vi "_PC_Daemon_DisInstrumentParam.vi"(8 "error in":errorcluster, 11 "ExpCondi":T1=[{"Label"="Laser", "Value"=variant}, {"Label"="Pressure", "Value"=variant}, {"Label"="TMP", "Value"=variant}, {"Label"="Script", "Value"=variant}, {"Label"="Signal Remarks", "Value"=variant}, {"Label"="ExtAO", "Value"=variant}, {"Label"="ExtDO", "Value"=variant}, {"Label"="ExtDI", "Value"=variant}, {"Label"="D999", "Value"=variant}]) -> (0 "error out":errorcluster)   [LabVIEW 2018]
uses:
  RT/PublicSubVI/Ctl/_ctl_RT_ExpCondi.ctl
  <vilib>/Utility/miscctls.llb/LVRowAndColumnTypeDef.ctl
  <vilib>/Utility/miscctls.llb/LVRowAndColumnUnsignedTypeDef.ctl
  <vilib>/event_ctls.llb/eventvkey.ctl
  PublicSubVI/Ctl/RegistyFunc.ctl
  <vilib>/Utility/file.llb/Write Delimited Spreadsheet (string).vi
panel:
  in  "Close Button":bool
  in  "Export Button":bool
  out "Table":string[][](table)
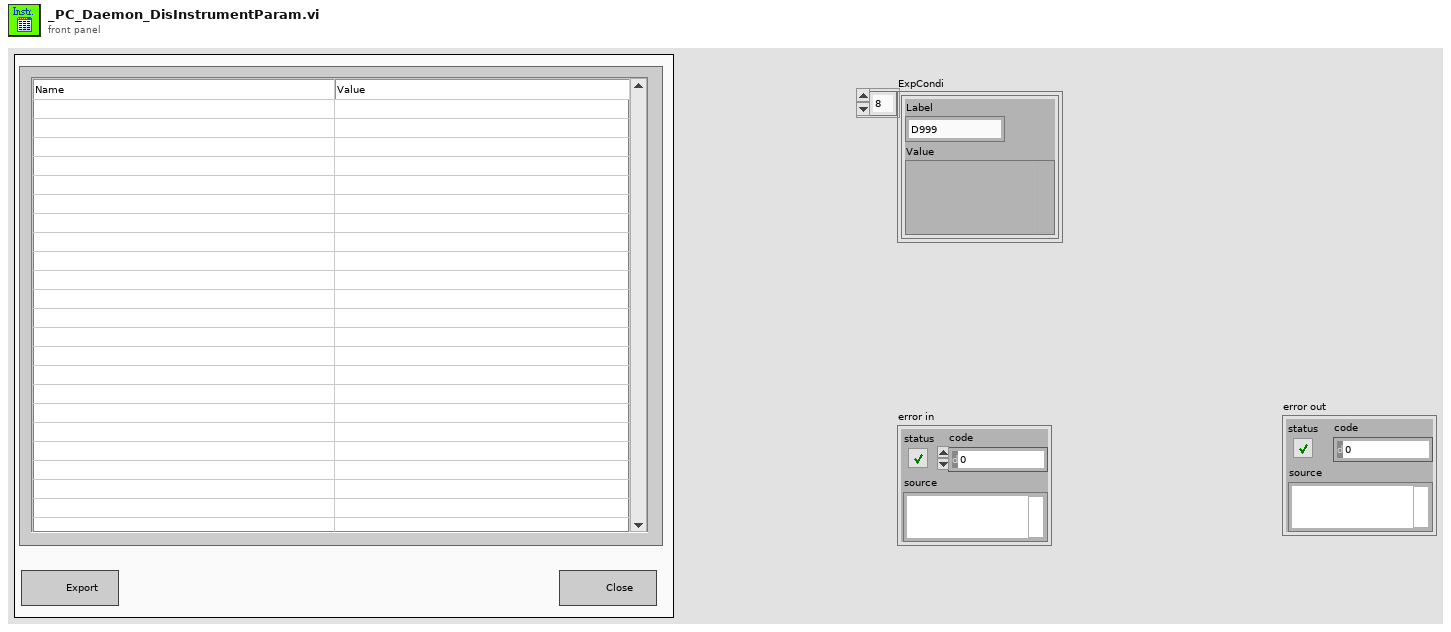
[diagram p1: front panel]
types:
  T1 = typedef "_ctl_RT_ExpCondi.ctl" = cluster{"Label":string, "Value":variant}[]
  T2 = typedef "LVRowAndColumnUnsignedTypeDef.ctl" = cluster{"Row":u32, "Column":u32}
  T3 = typedef "LVRowAndColumnTypeDef.ctl" = cluster{"Row":i32, "Column":i32}
  T4 = typedef "eventvkey.ctl" = enum16{"ASCII", "Enter", "Return", "Shift", "Ctrl", "Alt", "Cmd", "Opt", "Caps", "NumLock", "Clear", "Break", "Up", "Down", "Left", "Right", "Insert", "Delete", "Home", "End", "PageUp", "PageDown", "Escape", "Help", "Pause", "ScrollLock", "F1", "F2", "F3", "F4", "F5", "F6", "F7", "F8", "F9", "F10", "F11", "F12", "F13", "F14", "F15", "F16", "F17", "F18", "F19", "F20", "F21", "F22", "F23", "F24", "Play", "VolumeUp", "VolumeDown", "Mute", "Two Byte Char"}
  T5 = typedef "RegistyFunc.ctl" = enum16{"None", "FileAutoSave", "FileNoise", "FileSN", "ExeStatu", "WorkFolderPath", "MethodPath", "AVGItem", "LoopItem", "AutoRun", "BGColor", "LineColor", "LineWidth", "XGrid", "YGrid", "DeviceRefnum"}
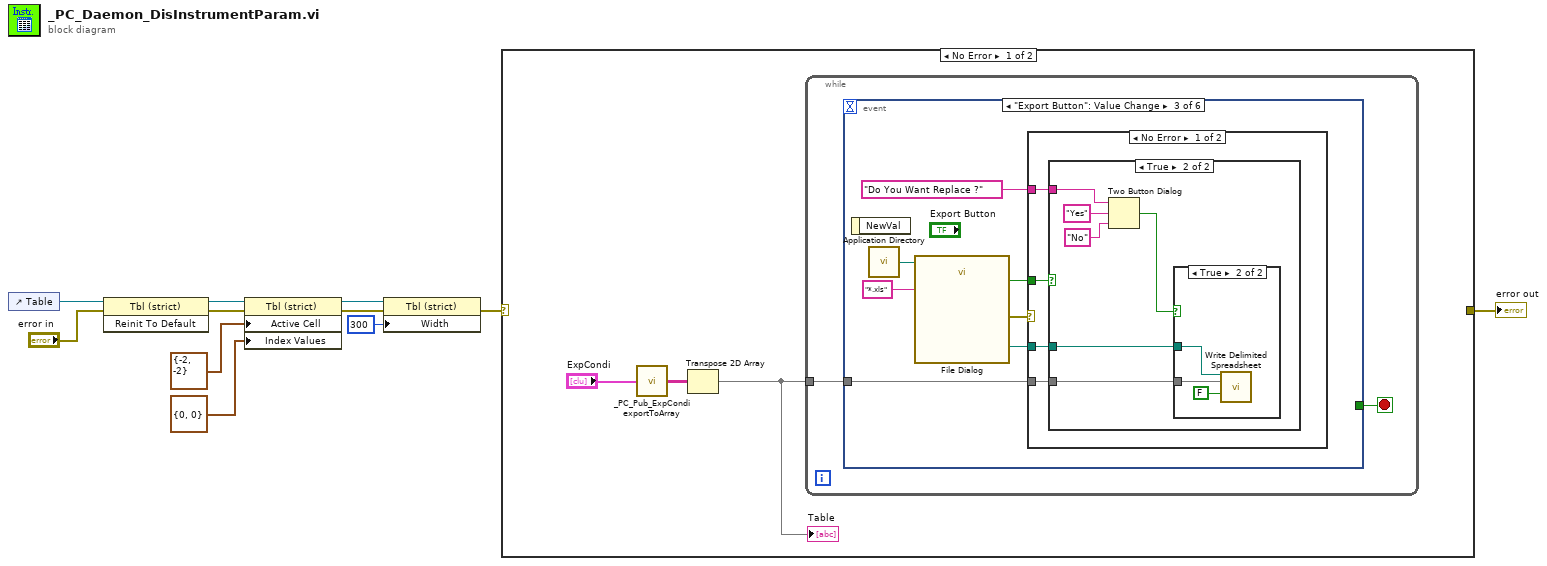
[diagram p0: block diagram]
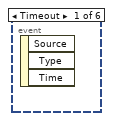
[diagram p2: hidden frame]
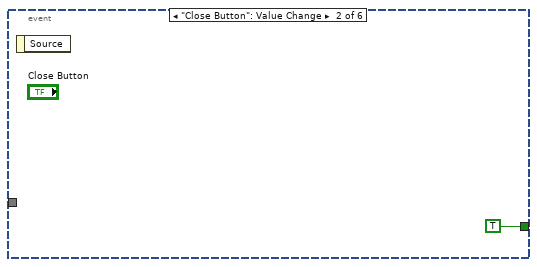
[diagram p3: hidden frame]
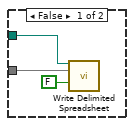
[diagram p4: hidden frame]
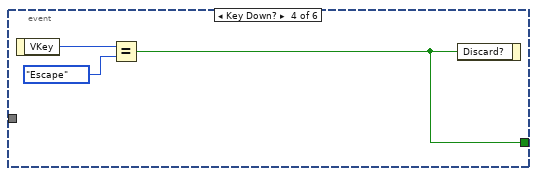
[diagram p7: hidden frame]
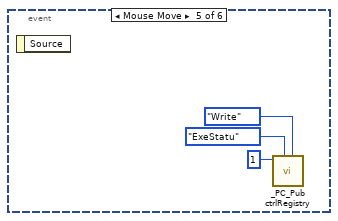
[diagram p8: hidden frame]
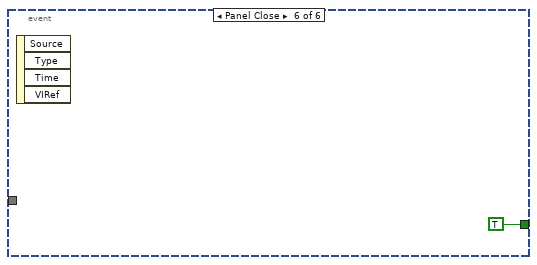
[diagram p9: hidden frame]
diagram:
  n1 = control-ref of="Table"() -> (w6:refnum<vi>)
  n2 = invoke class="Tbl (strict)" method="Reinit To Default"(reference=w6, error in="error in") -> (reference out=w5:refnum<vi>, error out=w4:errorcluster)  [unwired: 1 in, 1 out]
  n3 = property class="Tbl (strict)"(reference=w5, error in=w4, "Active Cell"=T3 {"Row"=-2, "Column"=-2} ("Active Cell:Active Cell"), "Index Values"=T2 {"Row"=0, "Column"=0}) -> (reference out=w9:refnum<vi>, error out=w8:errorcluster)
  n4 = property class="Tbl (strict)"(reference=w9, error in=w8, "Width"=u32 300 ("Active Cell:Cell Size:Width")) -> (error out=w2:errorcluster)  [unwired: 1 out]
  n5 = case shown="No Error" w2 {
    selector: w2 -> [_ w48]
    tunnel: [_ w48] -> w1
    frame No Error {
      n6 = call "_PC_Pub_ExpCondi exportToArray.vi"("ExpCondi"="ExpCondi") -> ("appended array"=w14:string[][])
      n7 = Transpose 2D Array(2D array=w14) -> (transposed array=w13:string[][])
      "Table" <- w13
      n8 = while {
        tunnel: w13 -> [w15]
        stop <- w16 stop-if-true
        n9 = event shown="[2] \"Export Button\": Value Change" {
          selector: _ -> [_ _ _ _ _ _]
          dyn-events: _ -> [_ _ _ _ _ _]
          timeout: _ -> [_ _ _ _ _ _]
          tunnel: [_ TRUE _ w41 _ TRUE] -> w16
          tunnel: w15 -> [_ _ w22 _ _ _]
          event Timeout {
            n10 = event-data() -> ()  [unwired: 1 in, 3 out]
          }
          event "Close Button": Value Change {
            n11 = event-data() -> ()  [unwired: 1 in, 1 out]
          }
          event "Export Button": Value Change {
            n12 = event-data() -> ()  [unwired: 1 in, 1 out]
            n13 = call <vilib>:"Application Directory.vi"() -> ("Application Directory"=w24:path)
            n14 = call "File Dialog"("start path"=w24, "pattern (all files)"="*.xls") -> ("selected path"=w23:path, "exists"=w19:bool, "error out"=w20:errorcluster)  [unwired: 10 in, 1 out]
            n15 = case shown="No Error" w20 {
              tunnel: w23 -> [w28 _]
              tunnel: w22 -> [w27 _]
              tunnel: w19 -> [w26 _]
              tunnel: "Do You Want Replace ?" ("T button name (\"OK\")") -> [w25 _]
              frame No Error {
                n16 = case shown="True" w26 {
                  tunnel: w28 -> [w30 w37]
                  tunnel: w27 -> [w29 w36]
                  tunnel: w25 -> [_ w33]
                  frame False {
                    n17 = call-poly <vilib>:"Write Delimited Spreadsheet.vi"("file path (dialog if empty)"=w30, "2D data"=w29, "append to file? (new file:F)"=FALSE) -> ()  [unwired: 11 in, 2 out]
                  }
                  frame True {
                    n18 = Two Button Dialog(message=w33, 1:"No" ("F button name (\"Cancel\")"), 2:"Yes" ("T button name (\"OK\")")) -> (T button?=w32:bool)
                    n19 = case shown="True" w32 {
                      tunnel: w37 -> [_ w40]
                      tunnel: w36 -> [_ w39]
                      frame False {
                      }
                      frame True {
                        n20 = call-poly <vilib>:"Write Delimited Spreadsheet.vi"("file path (dialog if empty)"=w40, "2D data"=w39, "append to file? (new file:F)"=FALSE) -> ()  [unwired: 11 in, 2 out]
                      }
                    }
                  }
                }
              }
              frame Error {
              }
            }
          }
          event Key Down? {
            n21 = event-data() -> ("VKey"=w43:T4)  [unwired: 1 in]
            n22 = Equal?(x=w43, y=eventvkey."Escape") -> (x = y?=w41:bool)
            n23 = event-data("Discard?"=w41) -> ()  [unwired: 1 in, 1 out]
          }
          event Mouse Move {
            n24 = event-data() -> ()  [unwired: 1 in, 1 out]
            n25 = call "_PC_Pub ctrlRegistry.vi"("type"=enum16{"None", "Write", "Read"}."Write", "function"=RegistyFunc."ExeStatu", "write value"=u32 1) -> ()  [unwired: 5 in, 4 out]
          }
          event Panel Close {
            n26 = event-data() -> ()  [unwired: 1 in, 4 out]
          }
        }
      }
    }
    frame Error {
    }
  }
  "error out" <- w1
